vi "rsrtx_FormatARINCWordRepCapInt_ReadCallback.vi"(5 "Attribute":T1={"Identifier"="", "Descriptive Name"="", "Data Type"=enum."Integer 32", "Command"="", "Access"=enum."Read/Write", "Range Table"="", "Read Callback"="", "Write Callback"="", "Supported Models"="", "Instrument Options"="", "Index"=0, "OPC Wait"=FALSE, "No Status Check"=FALSE, "Cache Only"=FALSE}, 7 "Repeated Capability":string, 8 "error in":errorcluster caption="error in (no error)", 11 "VISA resource name":refnum<visa-resource-name>) -> (0 "error out":errorcluster, 2 "Attribute Value I32":i32, 3 "VISA resource name out":refnum<visa-resource-name>)   [LabVIEW 2020, in "Rohde&Schwarz RTx Oscilloscopes.lvlib"]
doc: "This VI sets the attribute value.\n\nThis is a low-level VI that you can use to set the values of instrument-specific properties and inherent IVI properties. If the property represents an instrument state, this VI performs instrument I/O in the following cases:\n\n- State caching is disabled for the entire session or for the particular property.\n\n- State caching is enabled and the currently cached value is invalid or is different than the value you specify. \n\nThis instrument driver contains high-level VIs that set most of the instrument properties. It is best to use the high-level driver VIs as much as possible. They handle order dependencies and multithread locking for you. In addition, they perform status checking only after setting all of the properties. In contrast, when you set multiple properties using the SetAttribute VIs, the VIs check the instrument status after each call.\n\nAlso, when state caching is enabled, the high-level VIs that configure multiple properties perform instrument I/O only for the properties whose value you change. Thus, you can safely call the high-level VIs without the penalty of redundant instrument I/O."
uses:
  Rohde&Schwarz RTx Oscilloscopes.lvlib
  type_Attribute.ctl
  type_Attribute_Data_Type.ctl
  type_ReadWriteAccess.ctl
  rsidr_core.lvlib
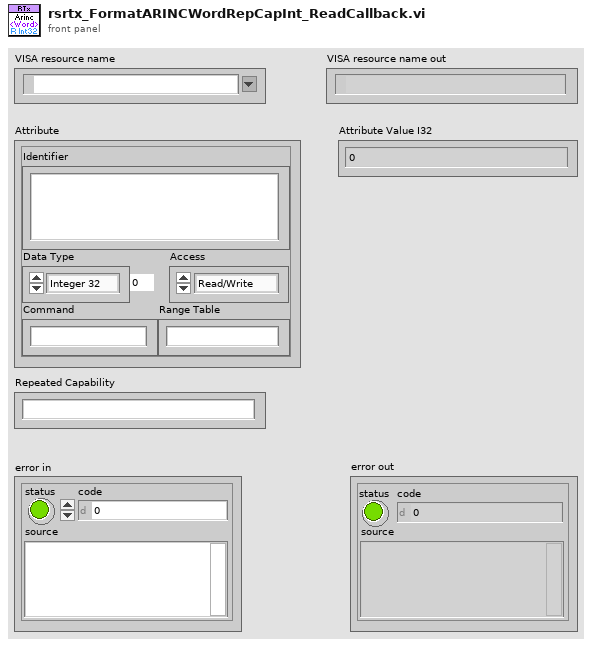
[diagram p1: front panel]
types:
  T1 = typedef "Rohde&Schwarz RTx Oscilloscopes.lvlib/rsidr_core.lvlib/type_Attribute.ctl" = cluster{"Identifier":string, "Descriptive Name":string, "Data Type":T2, "Command":string, "Access":T3, "Range Table":string, "Read Callback":string, "Write Callback":string, "Supported Models":string, "Instrument Options":string, "Index":i32, "OPC Wait":bool, "No Status Check":bool, "Cache Only":bool}
  T2 = typedef "Rohde&Schwarz RTx Oscilloscopes.lvlib/rsidr_core.lvlib/type_Attribute_Data_Type.ctl" = enum16{"Integer 32", "Double", "String", "Boolean", "None", "Integer 64", "RawString"}
  T3 = typedef "Rohde&Schwarz RTx Oscilloscopes.lvlib/rsidr_core.lvlib/type_ReadWriteAccess.ctl" = enum16{"Read Only", "Write Only", "Read/Write"}
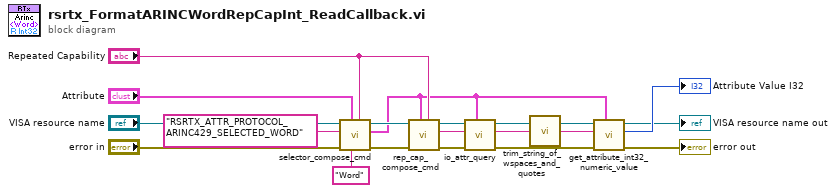
[diagram p0: block diagram]
diagram:
  n1 = call "selector_compose_cmd.vi"("Repeated Capability"="Repeated Capability", "Selector Name"="Word" ("search string"), "Attribute"="Attribute", "error in"="error in", "Selector Attribute ID"="RSRTX_ATTR_PROTOCOL_ARINC429_SELECTED_WORD", "VISA resource name"="VISA resource name") -> ("error out"=w16:errorcluster, "Attribute out"=w1:T1, "VISA resource name out"=w15:refnum<visa-resource-name>)  [unwired: 3 in]
  n2 = call "rep_cap_compose_cmd.vi"("Repeated Capability"="Repeated Capability", "Attribute"=w1, "error in"=w16, "VISA resource name"=w15) -> ("error out"=w14:errorcluster, "Command out"=w19:string, "VISA resource name out"=w13:refnum<visa-resource-name>)  [unwired: 5 in]
  n3 = call "io_attr_query.vi"("Attribute"=w1, "error in"=w14, "write buffer"=w19, "VISA resource name"=w13) -> ("error out"=w5:errorcluster, "read buffer"=w7:string, "VISA resource name out"=w4:refnum<visa-resource-name>)  [unwired: 5 in]
  n4 = call "trim_string_of_wspaces_and_quotes.vi"("String in"=w7) -> ("String out"=w6:string)  [unwired: 4 in]
  n5 = call "get_attribute_int32_numeric_value.vi"("Attribute"=w1, "error in"=w5, "Cmd Value in"=w6, "VISA resource name"=w4) -> ("error out"=→"error out":errorcluster, "Int32 value out"=→"Attribute Value I32":i32, "VISA resource name out"=→"VISA resource name out":refnum<visa-resource-name>)  [unwired: 5 in]
